vi "Align.vi"() -> ()   [LabVIEW 2012]
uses:
  Madlib.dll
panel:
  out "Read Theta C":dbl format="%.3f"
  out "Read Theta B":dbl format="%.3f"
  out "Read Theta A":dbl format="%.3f"
  in  "?":bool
  out "Width (mm)":dbl format="%.2f"
  out "Height (mm)":dbl format="%.2f"
  in  "C":dbl format="%.3f"
  in  "B":dbl format="%.3f"
  in  "Theta A":dbl caption="A" format="%.3f"
  # "Command"
  # "Position"
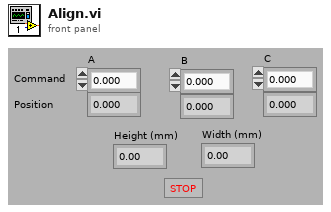
[diagram p1: front panel]
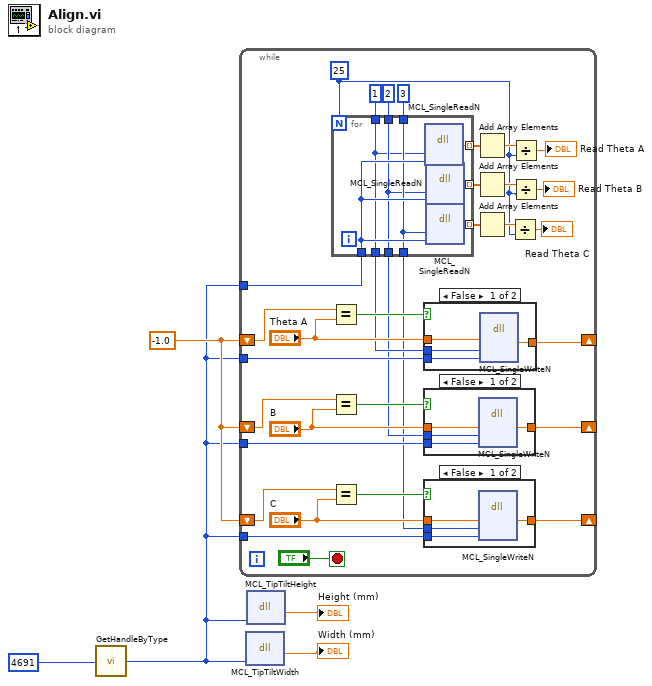
[diagram p0: block diagram]
diagram:
  w3 = -1.0
  n1 = call "GetHandleByType.vi"("Type"=4691) -> ("Handle"=w2:i32)
  n2 = while {
    shift-right: [w35] -> _
    shift-left: w3 -> [w38]
    shift-right: [w34] -> _
    shift-left: w3 -> [w37]
    shift-right: [w33] -> _
    shift-left: w3 -> [w36]
    tunnel: w2 -> [w26]
    tunnel: w2 -> [w25]
    tunnel: w2 -> [w24]
    tunnel: w2 -> [w19]
    stop <- "?" stop-if-true
    w9 = 25
    n3 = Equal?(x=w38, y="Theta A") -> (x = y?=w27:bool)
    n4 = Equal?(x=w37, y="B") -> (x = y?=w32:bool)
    n5 = Equal?(x=w36, y="C") -> (x = y?=w31:bool)
    n6 = for {
      N: w9 -> [_]
      tunnel: [w39] -> w22
      tunnel: [w40] -> w21
      tunnel: [w41] -> w20
      tunnel: w19 -> [w45]
      tunnel: [w44] -> w14 mode=indexing
      tunnel: [w43] -> w15 mode=indexing
      tunnel: [w42] -> w13 mode=indexing
      tunnel: 3 -> [w41]
      tunnel: 2 -> [w40]
      tunnel: 1 -> [w39]
      n7 = dll-call lib="C:/Users/Labview/Desktop/SRR/Madlib_x64/Labview Examples/MADLib.dll" fn="MCL_SingleReadN"("axis"=w39, "handle"=w45) -> (w44:dbl)  [unwired: 5 in, 2 out]
      n8 = dll-call lib="C:/Users/Labview/Desktop/SRR/Madlib_x64/Labview Examples/MADLib.dll" fn="MCL_SingleReadN"("axis"=w40, "handle"=w45) -> (w43:dbl)  [unwired: 5 in, 2 out]
      n9 = dll-call lib="C:/Users/Labview/Desktop/SRR/Madlib_x64/Labview Examples/MADLib.dll" fn="MCL_SingleReadN"("axis"=w41, "handle"=w45) -> (w42:dbl)  [unwired: 5 in, 2 out]
    }
    n10 = case shown="False" w27 {
      tunnel: [w59 w60] -> w35
      tunnel: "Theta A" -> [w58 w60]
      tunnel: w26 -> [w57 _]
      tunnel: w22 -> [w56 _]
      frame False {
        n11 = dll-call lib="C:/Users/Labview/Desktop/SRR/Madlib_x64/Labview Examples/MADLib.dll" fn="MCL_SingleWriteN"("position"=w58, "axis"=w56, "handle"=w57) -> ("position"=w59:dbl)  [unwired: 6 in, 2 out]
      }
      frame True {
      }
    }
    n12 = case shown="False" w32 {
      tunnel: [w54 w55] -> w34
      tunnel: "B" -> [w53 w55]
      tunnel: w25 -> [w52 _]
      tunnel: w21 -> [w51 _]
      frame False {
        n13 = dll-call lib="C:/Users/Labview/Desktop/SRR/Madlib_x64/Labview Examples/MADLib.dll" fn="MCL_SingleWriteN"("position"=w53, "axis"=w51, "handle"=w52) -> ("position"=w54:dbl)  [unwired: 6 in, 2 out]
      }
      frame True {
      }
    }
    n14 = case shown="False" w31 {
      tunnel: [w49 w50] -> w33
      tunnel: "C" -> [w48 w50]
      tunnel: w24 -> [w47 _]
      tunnel: w20 -> [w46 _]
      frame False {
        n15 = dll-call lib="C:/Users/Labview/Desktop/SRR/Madlib_x64/Labview Examples/MADLib.dll" fn="MCL_SingleWriteN"("position"=w48, "axis"=w46, "handle"=w47) -> ("position"=w49:dbl)  [unwired: 6 in, 2 out]
      }
      frame True {
      }
    }
    n16 = Add Array Elements(numeric array=w14) -> (sum=w12:dbl)
    n17 = Add Array Elements(numeric array=w15) -> (sum=w11:dbl)
    n18 = Add Array Elements(numeric array=w13) -> (sum=w10:dbl)
    n19 = Divide(x=w10, y=w9) -> (x/y=→"Read Theta C":dbl)
    n20 = Divide(x=w12, y=w9) -> (x/y=→"Read Theta A":dbl)
    n21 = Divide(x=w11, y=w9) -> (x/y=→"Read Theta B":dbl)
  }
  n22 = dll-call lib="C:/Users/Labview/Desktop/SRR/Madlib_x64/Labview Examples/MADLib.dll" fn="MCL_TipTiltWidth"("handle"=w2) -> (→"Width (mm)":dbl)  [unwired: 4 in, 2 out]
  n23 = dll-call lib="C:/Users/Labview/Desktop/SRR/Madlib_x64/Labview Examples/MADLib.dll" fn="MCL_TipTiltHeight"("handle"=w2) -> (→"Height (mm)":dbl)  [unwired: 4 in, 2 out]
